vi "Configure Multi Eval Meas Limit ACLR.vi"(0 "VISA resource name":refnum<visa-resource-name>, 1 "Relative Level Enabled (Off)":i32(ring) items=["Off", "On", "Value"], 2 "Absolute Level Enabled (Off)":i32(ring) items=["Off", "On", "Value"], 5 "Instance (1)":T3=1, 7 "Bandwidth (50 MHz)":T2 items=["50 MHz", "100 MHz", "200 MHz", "400 MHz"], 9 "Limit Band (Band n257, n258, n261)":T1=1 items=["Band n257, n258, n261"=1, "Bands n260"=2], 11 "error in (no error)":errorcluster, 12 "Relative Level (18.0)":dbl=18.0 format="%^.3e", 13 "Absolute Level (-35.0)":dbl=-35.0 format="%^.3e") -> (4 "VISA resource name out":refnum<visa-resource-name>, 15 "error out":errorcluster)   [LabVIEW 2020, in "Rohde&Schwarz CMXP NR FR2 Measurement.lvlib"]
doc: "Defines relative and absolute limits for the ACLR measured in an adjacent NR channel. The settings are defined separately for each channel bandwidth.\n\nAttribute:\nRSCMXPNRFR2M_ATTR_MULTI_EVAL_MEASUREMENT_LIMIT_ACLR\n\nRemote-control command:\nCONFigure:NRMMw:MEAS<i>:MEValuation:LIMit:ACLR:NR:CBANdwidth<bw>:BLIMits<n>"
uses:
  <instrlib>/Rohde&Schwarz CMXP NR FR2 Measurement/Rohde&Schwarz CMXP NR FR2 Measurement.lvlib
  <instrlib>/Rohde&Schwarz CMXP NR FR2 Measurement/Private/_Instance.ctl
  <instrlib>/Rohde&Schwarz CMXP NR FR2 Measurement/Private/_Bandwidth.ctl
  <instrlib>/Rohde&Schwarz CMXP NR FR2 Measurement/Private/_Limit Band.ctl
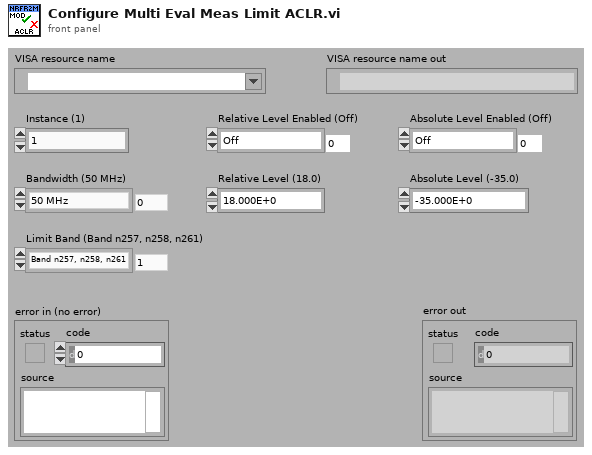
[diagram p1: front panel]
types:
  T1 = typedef "Rohde&Schwarz CMXP NR FR2 Measurement.lvlib/_Limit Band.ctl" = i32
  T2 = typedef "Rohde&Schwarz CMXP NR FR2 Measurement.lvlib/_Bandwidth.ctl" = i32
  T3 = typedef "Rohde&Schwarz CMXP NR FR2 Measurement.lvlib/_Instance.ctl" = i32
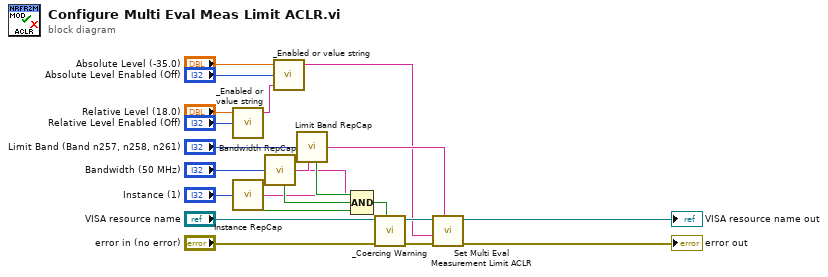
[diagram p0: block diagram]
diagram:
  n1 = call <instrlib>:"_Enabled or value string.vi"("Enabled or Value"="Relative Level Enabled (Off)", "Value"="Relative Level (18.0)") -> ("Resulting String"=w11:string)  [unwired: 3 in]
  n2 = call <instrlib>:"Instance RepCap.vi"("Instance In"="Instance (1)") -> ("In Range?"=w18:bool, "RepCap Identifier Out"=w2:string)  [unwired: 1 in]
  n3 = call <instrlib>:"Bandwidth RepCap.vi"("Bandwidth In"="Bandwidth (50 MHz)", "RepCap String In (\"\")"=w2) -> ("In Range?"=w17:bool, "RepCap Identifier Out"=w16:string)
  n4 = call <instrlib>:"_Enabled or value string.vi"("Initial String"=w11, "Enabled or Value"="Absolute Level Enabled (Off)", "Value"="Absolute Level (-35.0)") -> ("Resulting String"=w1:string)  [unwired: 2 in]
  n5 = call <instrlib>:"Limit Band RepCap.vi"("Limit Band In"="Limit Band (Band n257, n258, n261)", "RepCap String In (\"\")"=w16) -> ("In Range?"=w15:bool, "RepCap Identifier Out"=w6:string)
  n6 = Compound Arithmetic op=AND(w15, w17, w18) -> (w9:bool)
  n7 = call <instrlib>:"_Coercing Warning.vi"("In Range?"=w9, "error in (no error)"="error in (no error)", "VISA resource name"="VISA resource name") -> ("error out"=w7:errorcluster, "VISA resource name out"=w8:refnum<visa-resource-name>)  [unwired: 7 in]
  n8 = call "Set Multi Eval Measurement Limit ACLR"("Repeated Capabilities"=w6, "error in (no error)"=w7, "Multi Eval Measurement Limit ACLR ()"=w1, "instrument handle"=w8) -> ("error out"=→"error out":errorcluster, "instrument handle out"=→"VISA resource name out":refnum<visa-resource-name>)  [unwired: 6 in]
